vi "ziGetValueDouble.vi"(3 "error in":errorcluster, 4 "Path":string, 5 "Handle in":T1 {"Handle" format="0x%08x"; "Conn" format="0x%08x"}) -> (0 "error out":errorcluster, 1 "Value":dbl, 2 "Handle out":T1 {"Handle" format="0x%08x"; "Conn" format="0x%08x"})   [LabVIEW 2019, in "Zurich Instruments LabOne.lvlib"]
doc: "This vi retrieves the numerical value of the specified node as an double-type value. The vi returns the value first found that matches Path if more than one value is available (a wildcard is used in the Path)."
uses:
  Zurich Instruments LabOne.lvlib
  ziTypeHandle.ctl
  Private/ziLV64.dll
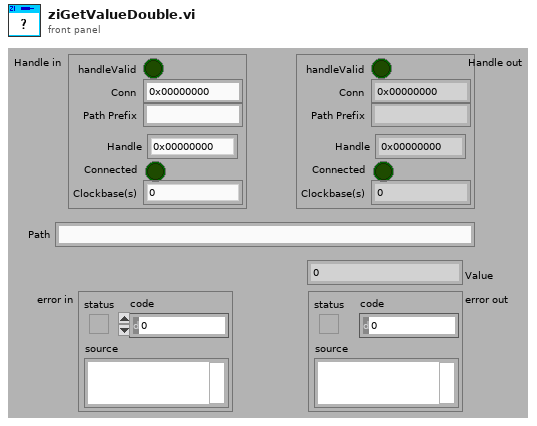
[diagram p1: front panel]
types:
  T1 = typedef "Zurich Instruments LabOne.lvlib/ziTypeHandle.ctl" = cluster{"handleValid":bool, "Conn":u64, "Path Prefix":string, "Handle":u64, "Connected":bool, "Clockbase(s)":dbl}
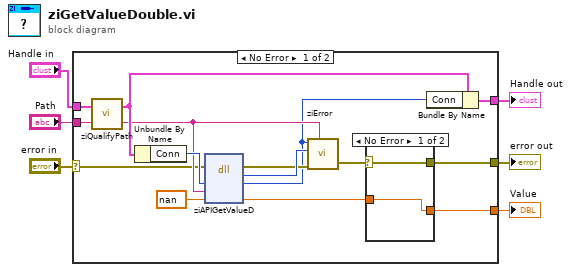
[diagram p0: block diagram]
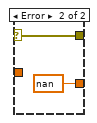
[diagram p2: hidden frame]
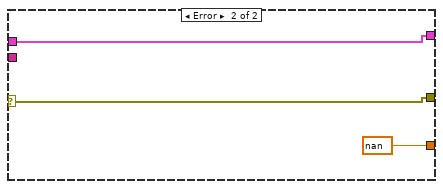
[diagram p3: hidden frame]
diagram:
  n1 = case shown="No Error" "error in" {
    selector: "error in" -> [w12 w28]
    tunnel: [w7 nan ("Value")] -> w6
    tunnel: [w9 w28] -> w5
    tunnel: [w18 w27] -> w4
    tunnel: "Handle in" -> [w17 w27]
    tunnel: "Path" -> [w16 _]
    frame No Error {
      n2 = call "ziQualifyPath.vi"("Path In"=w16, "Handle In"=w17) -> ("Path Out"=w14:string, "Handle Out"=w15:T1)
      n3 = Unbundle By Name(w15) -> ("Conn"=w21:u64)
      n4 = dll-call lib="G:/01_software/CryoTUM/sub_vi-s/Equipment/Zurich Instruments LabOne/Private/ziLV*.*" fn="ziAPIGetValueD"(error in=w12, "Conn"=w21, "Path"=w14, "Value"=nan) -> (error out=w19:errorcluster, "return type"=w20:u32, "Conn"=w13:u64, "Value"=w8:dbl)  [unwired: 2 in, 2 out]
      n5 = call "ziError.vi"("Conn"=w13, "ziErrorCode"=w20, "Error In"=w19, "Annotation"=w14) -> ("Error Out"=w10:errorcluster)  [unwired: 1 in, 1 out]
      n6 = case shown="No Error" w10 {
        selector: w10 -> [w23 w25]
        tunnel: [w23 w25] -> w9
        tunnel: w8 -> [w22 _]
        tunnel: [w22 nan ("Value")] -> w7
        frame No Error {
        }
        frame Error {
        }
      }
      n7 = Bundle By Name(cluster=w15, "Conn"=w13) -> (w18:T1)
    }
    frame Error {
    }
  }
  "Handle out" <- w4
  "error out" <- w5
  "Value" <- w6
